vi "SetShutterModes.vi"(8 "error in (no error)":errorcluster, 10 "Shutters":T1, 11 "Operational Mode":T3) -> (0 "error out":errorcluster, 2 "Shutters Out":T1, 3 "Operational Mode Out":T3)   [LabVIEW 2016]
uses:
  Controls/Operational Modes.ctl
  Controls/Shutters.ctl
  Controls/Shutter Data.ctl
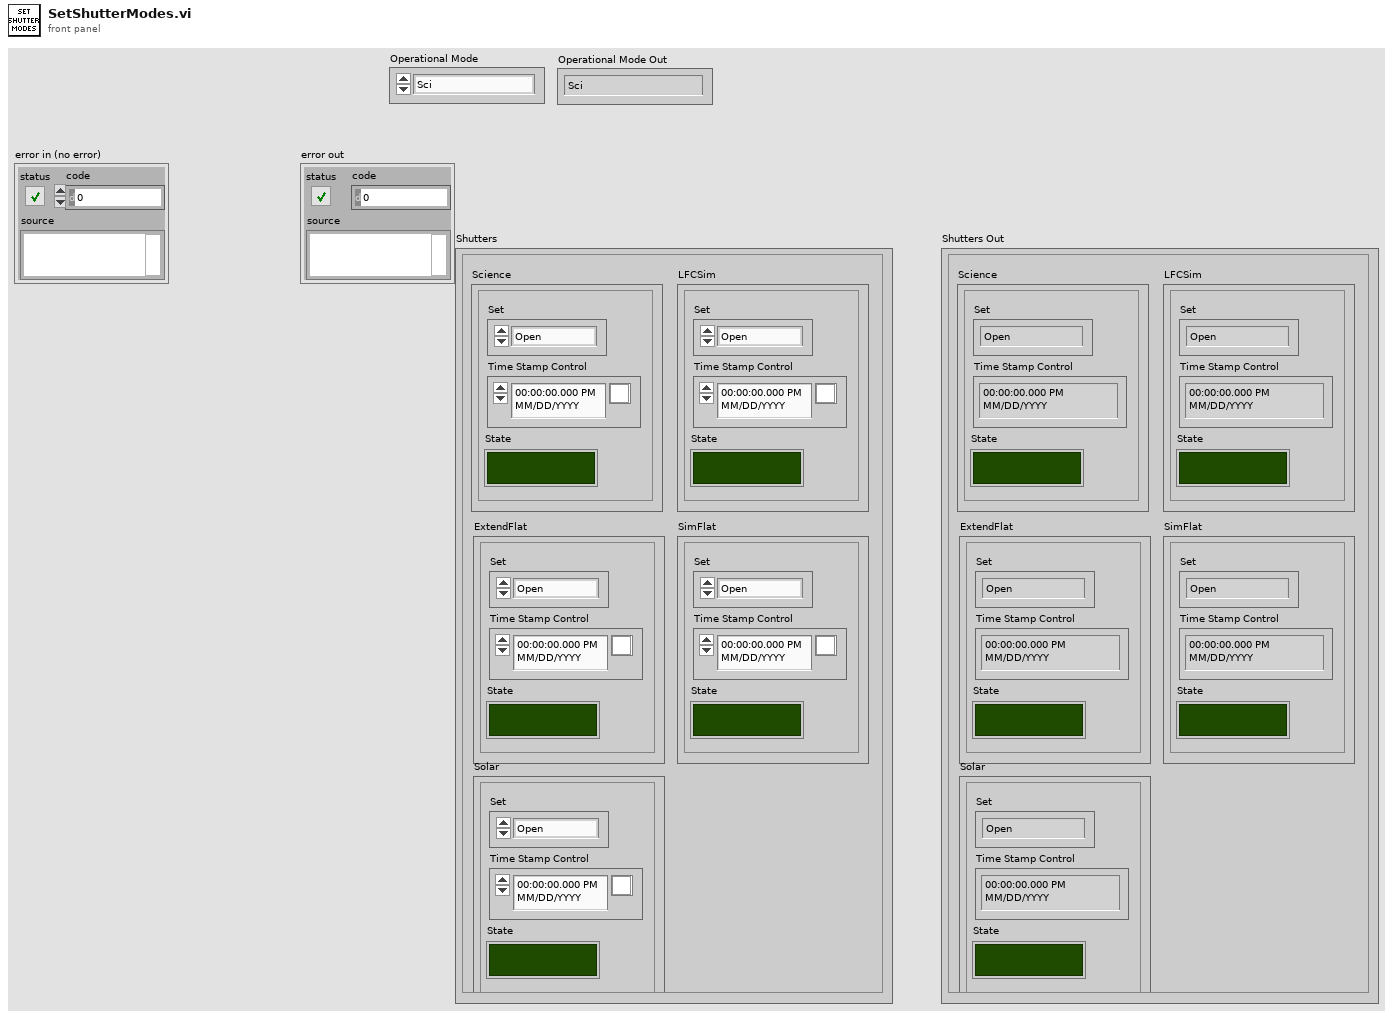
[diagram p1: front panel]
types:
  T1 = typedef "Shutters.ctl" = cluster{"Science":T2, "LFCSim":T2, "ExtendFlat":T2, "SimFlat":T2, "Solar":T2}
  T2 = typedef "Shutter Data.ctl" = cluster{"Set":enum16{"Open", "Close", "Arm", "Idle"}, "Time Stamp Control":timestamp, "State":bool}
  T3 = typedef "Operational Modes.ctl" = enum16{"Sci", "Sci-Sim", "Solar", "Solar-Sim", "LFC-Sci", "LFC-Sim", "LFC-Both", "ThAr", "ThAr-Sim", "Flat", "ExtFlat", "ExtFlat-Sim", "ExtFlat-Both", "Qtz", "ExtQtz", "ExtQtz-Sim", "ExtQtz-Both", "Dark"}
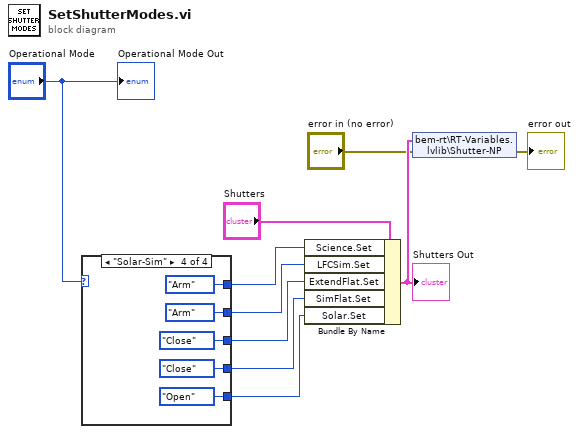
[diagram p0: block diagram]
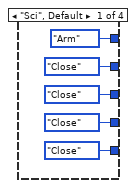
[diagram p2: hidden frame]
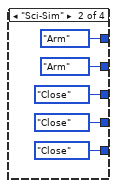
[diagram p3: hidden frame]
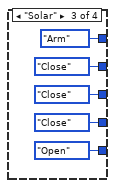
[diagram p4: hidden frame]
diagram:
  n1 = case shown="\"Solar-Sim\"" "Operational Mode" {
    tunnel: [enum16{"Open", "Close", "Arm", "Idle"}."Arm" ("LFCSim.Set") enum16{"Open", "Close", "Arm", "Idle"}."Arm" ("LFCSim.Set") enum16{"Open", "Close", "Arm", "Idle"}."Arm" ("LFCSim.Set") enum16{"Open", "Close", "Arm", "Idle"}."Arm" ("LFCSim.Set")] -> w9
    tunnel: [enum16{"Open", "Close", "Arm", "Idle"}."Close" ("Science.Set") enum16{"Open", "Close", "Arm", "Idle"}."Arm" ("Science.Set") enum16{"Open", "Close", "Arm", "Idle"}."Close" ("Science.Set") enum16{"Open", "Close", "Arm", "Idle"}."Arm" ("Science.Set")] -> w8
    tunnel: [enum16{"Open", "Close", "Arm", "Idle"}."Close" ("ExtendFlat.Set") enum16{"Open", "Close", "Arm", "Idle"}."Close" ("ExtendFlat.Set") enum16{"Open", "Close", "Arm", "Idle"}."Close" ("ExtendFlat.Set") enum16{"Open", "Close", "Arm", "Idle"}."Close" ("ExtendFlat.Set")] -> w7
    tunnel: [enum16{"Open", "Close", "Arm", "Idle"}."Close" ("Solar.Set") enum16{"Open", "Close", "Arm", "Idle"}."Close" ("Solar.Set") enum16{"Open", "Close", "Arm", "Idle"}."Close" ("Solar.Set") enum16{"Open", "Close", "Arm", "Idle"}."Close" ("Solar.Set")] -> w6
    tunnel: [enum16{"Open", "Close", "Arm", "Idle"}."Close" ("SimFlat.Set") enum16{"Open", "Close", "Arm", "Idle"}."Close" ("SimFlat.Set") enum16{"Open", "Close", "Arm", "Idle"}."Open" ("SimFlat.Set") enum16{"Open", "Close", "Arm", "Idle"}."Open" ("SimFlat.Set")] -> w5
    frame "Sci", Default {
    }
    frame "Sci-Sim" {
    }
    frame "Solar" {
    }
    frame "Solar-Sim" {
    }
  }
  n2 = Bundle By Name(cluster="Shutters", "Science.Set"=w9, "LFCSim.Set"=w8, "ExtendFlat.Set"=w7, "SimFlat.Set"=w6, "Solar.Set"=w5) -> (w3:T1)
  "Shutters Out" <- w3
  n3 = shared-variable "bem-rt\\RT-Variables.lvlib\\Shutter-NP"(w3, error in="error in (no error)") -> (error out=→"error out":errorcluster)
  "Operational Mode Out" <- "Operational Mode"
